vi "Get All Values By Enumerator.vi"(8 "error in (no error)":errorcluster caption="错误输入（无错误）", 11 "HashTable 输入":refnum<class "HashTable.lvclass"> caption="DNL_LabVIEW Object in") -> (0 "error out":errorcluster caption="错误输出", 2 "Values":variant[](array[variant]), 3 "HashTable 输出":refnum<class "HashTable.lvclass"> caption="DNL_LabVIEW Object out")   [LabVIEW 2012, in "HashTable.lvclass"]
uses:
  HashTable.lvclass
  Enumerator/Enumerator.lvclass
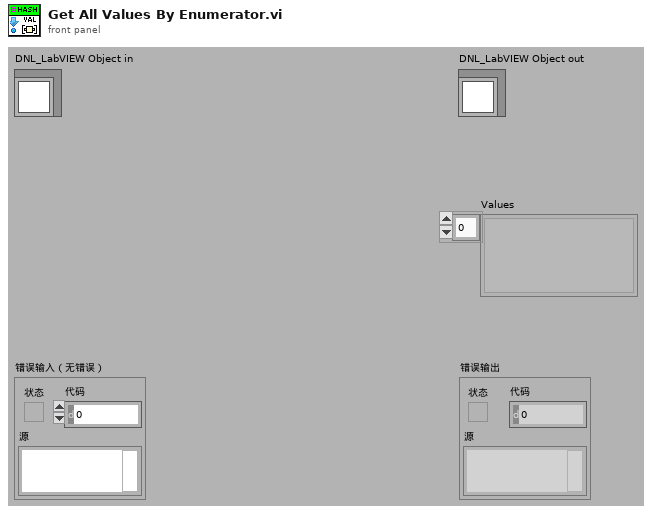
[diagram p1: front panel]
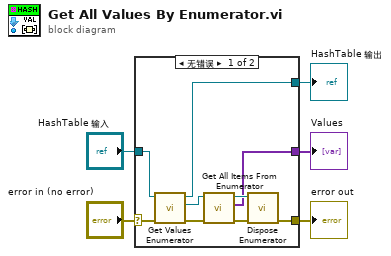
[diagram p0: block diagram]
diagram:
  n1 = case shown="无错误" "error in (no error)" {
    selector: "error in (no error)" -> [w10 w16]
    tunnel: [w11 w16] -> w4
    tunnel: [w7 w15] -> w2
    tunnel: "HashTable 输入" -> [w8 w15]
    tunnel: [w13 _] -> w1
    frame No Error {
      n2 = call "Get Values Enumerator.vi"("error in (no error)"=w10, "HashTable 输入"=w8) -> ("error out"=w9:errorcluster, "Enumerator 输出"=w6:refnum<class "Enumerator.lvclass">, "HashTable 输出"=w7:refnum<class "HashTable.lvclass">)  [unwired: 7 in]
      n3 = call "Get All Items From Enumerator.vi"("error in (no error)"=w9, "Enumerator 输入"=w6) -> ("error out"=w12:errorcluster, "Items"=w13:variant[], "Enumerator 输出"=w14:refnum<class "Enumerator.lvclass">)  [unwired: 7 in]
      n4 = call "Dispose Enumerator.vi"("error in (no error)"=w12, "Enumerator 输入"=w14) -> ("error out"=w11:errorcluster)  [unwired: 8 in, 1 out]
    }
    frame Error {
    }
  }
  "error out" <- w4
  "HashTable 输出" <- w2
  "Values" <- w1
